vi "HFRR ADV v09.vi"() -> ()   [LabVIEW 2025] (continued)
            n4154 = property class="Instr"(reference=w5657, error in=w5636) -> (reference out=w5656:refnum<visa-resource-name>, error out=w5655:errorcluster, "Serial Settings:Number of Bytes at Serial Port"=w5654:u32)
            n4155 = Greater?(x=w5654, y=u32 100) -> (0:w5652:bool)
            n4156 = case shown="True" w5652 {
              tunnel: w5656 -> [w5695 w5720]
              tunnel: w5655 -> [w5694 w5719]
              tunnel: w5654 -> [_ w5718]
              tunnel: [w5695 w5717] -> w5642
              tunnel: [w5694 w5716] -> w5641
              tunnel: w5638 -> [w5693 w5715]
              tunnel: [w5693 ""] -> w5637
              frame False {
              }
              frame True {
                w5705 = u32 6 ("y")
                # "Page 84 of \nmanual"
                n4157 = VISA Read(VISA resource name=w5720, byte count=w5718, error in (no error)=w5719) -> (VISA resource name out=w5717:refnum<visa-resource-name>, read buffer=w5713:string, error out=w5716:errorcluster)  [unwired: 1 out]
                n4158 = while {
                  tunnel: w5713 -> [w5769]
                  tunnel: [w5765] -> w5707 mode=indexing
                  tunnel: [w5759] -> w5711 mode=indexing
                  tunnel: [w5757] -> _
                  i -> [w5757]
                  stop <- w5762 stop-if-true
                  n4159 = String Subset(string=w5769, offset (0)=w5757) -> (substring=w5764:string)  [unwired: 1 in]
                  n4160 = String To Byte Array(string=w5764) -> (unsigned byte array=w5768:u8[])
                  n4161 = String Length(string=w5764) -> (length=w5763:i32)
                  n4162 = Index Array(array=w5768) -> (element=w5767:u8)  [unwired: 1 in]
                  n4163 = Equal To 0?(x=w5763) -> (x = 0?=w5762:bool)
                  n4164 = Number To Boolean Array(number=w5767) -> (Boolean array=w5761:bool[])
                  n4165 = Reverse 1D Array(array=w5761) -> (reversed array=w5760:bool[])
                  n4166 = And(x=w5761, y=bool[] [FALSE, FALSE, FALSE, FALSE, FALSE, FALSE, TRUE, TRUE] ("Boolean array")) -> (x .and. y?=w5765:bool[])
                  n4167 = And(x=w5760, y=bool[] [FALSE, FALSE, TRUE, TRUE, TRUE, TRUE, TRUE, TRUE] ("Boolean array")) -> (x .and. y?=w5759:bool[])
                }
                n4168 = Concatenate Strings(w5715, w5713) -> (→"Read String":string)
                n4169 = while {
                  tunnel: w5707 -> [w5756] mode=indexing
                  tunnel: [w5752] -> w5710
                  i -> [w5752]
                  stop <- w5753 stop-if-true
                  n4170 = Search 1D Array(1D array=w5756, element=TRUE) -> (index of element=w5754:i32)  [unwired: 1 in]
                  n4171 = Less Than 0?(x=w5754) -> (x < 0?=w5753:bool)
                }
                n4172 = Delete From Array(array=w5711, length=w5710, index (row)=0) -> (array with subset deleted=w5706:bool[][])  [unwired: 1 in, 1 out]
                n4173 = Array Size(array=w5706) -> (size(s)=w5708:i32[])
                n4174 = Index Array(array=w5708) -> (element=w5700:i32)  [unwired: 1 in]
                n4175 = Greater?(x=w5700, y=w5705) -> (0:w5703:bool)
                n4176 = Subtract(x=w5700, y=w5705) -> (x-y=w5704:u32)
                n4177 = Select(t=w5704, s=w5703, f=u32 0) -> (s? t:f=w5701:u32)
                n4178 = while {
                  tunnel: w5706 -> [w5739]
                  tunnel: [w5741] -> w5699 mode=indexing
                  tunnel: w5701 -> [w5723]
                  i -> [w5740]
                  stop <- w5738 stop-if-true
                  w5730 = 6 ("index")
                  w5729 = 2 ("length")
                  # "Page 65 of \nmanual"
                  n4179 = Multiply(x=u32 3 ("y"), y=w5740) -> (x*y=w5737:u32)
                  n4180 = Divide(x=u32 102 ("y"), y=u32 65520) -> (x/y=w5747:dbl)
                  n4181 = Greater Or Equal?(x=w5737, y=w5723) -> (x >= y?=w5738:bool)
                  n4182 = Index Array(array=w5739, index (row) #1=w5737) -> (element #1=w5735:bool[], element #2=w5734:bool[], element #3=w5733:bool[])  [unwired: 5 in]
                  n4183 = Reverse 1D Array(array=w5735) -> (reversed array=w5728:bool[])
                  n4184 = Reverse 1D Array(array=w5734) -> (reversed array=w5732:bool[])
                  n4185 = Reverse 1D Array(array=w5733) -> (reversed array=w5731:bool[])
                  n4186 = Delete From Array(array=w5728, length=w5729, index=w5730) -> (array with subset deleted=w5724:bool[])  [unwired: 1 out]
                  n4187 = Delete From Array(array=w5732, length=w5729, index=w5730) -> (array with subset deleted=w5725:bool[])  [unwired: 1 out]
                  n4188 = Delete From Array(array=w5731, length=w5729, index=w5730) -> (array with subset deleted=w5726:bool[])  [unwired: 1 out]
                  n4189 = Insert Into Array(array=bool[] [] ("Boolean array"), new element #1=w5724, new element #2=w5725, new element #3=w5726) -> (w5727:bool[])  [unwired: 1 in]
                  n4190 = Boolean Array To Number(Boolean array=w5727) -> (number=w5736:u32)
                  n4191 = Multiply(x=w5747, y=w5736) -> (x*y=w5746:dbl)
                  n4192 = Decrement(x=w5746) -> (x-1=w5745:dbl)
                  n4193 = Divide(x=w5745, y=u32 100) -> (x/y=w5743:dbl)
                  n4194 = Multiply(x=w5743, y=u32 10) -> (x*y=w5741:dbl)
                }
                n4195 = Delete From Array(array=w5699) -> (array with subset deleted=w5698:dbl[])  [unwired: 2 in, 1 out]
                "Waveform Graph 5" <- w5698
                "Waveform Chart 3" <- w5698
                n4196 = call-poly <vilib>:"Mean.vi"("X"=w5698) -> ("mean"=w5697:dbl)  [unwired: 1 out]
                "Measure_LDS" <- w5697
                n4197 = case shown="True" "Zero 4" {
                  tunnel: w5697 -> [_ w5722]
                  frame False {
                  }
                  frame True {
                    n4198 = local write "Zero 4"(FALSE ("Zero 4")) -> ()
                    "z_measure" <- w5722
                  }
                }
              }
            }
            n4199 = local read "Measure_LDS"() -> (w5632:dbl)
            n4200 = local read "Disp (mm)"() -> (w5631:dbl)
            n4201 = local read "Boolean 7"() -> (w5630:bool)
            n4202 = local read "Boolean 8"() -> (w5629:bool)
            n4203 = case shown="True" "Boolean 8" {
              tunnel: w5631 -> [_ w5662]
              tunnel: w5632 -> [_ w5661]
              frame False {
              }
              frame True {
                n4204 = local read "Captured Values 2"() -> (w5665:dbl[][])
                n4205 = Build Array(w5662, w5661) -> (w5660:dbl[])
                n4206 = Build Array (concatenate)(w5665, w5660) -> (w5663:dbl[][])
                n4207 = local write "Captured Values 2"(w5663) -> ()
                n4208 = local write "Boolean 8"(FALSE ("Boolean 8")) -> ()
              }
            }
            n4209 = call "Build XY Graph"("Enable"=w5629, "Reset"=w5630, "Y Input"=w5632, "X Input"=w5631) -> ("XY Graph"=→"?":cluster{"Y":dbl[], "Y":dbl[]}[])  [unwired: 6 in, 1 out]
            n4210 = case shown="True" "Boolean 9" {
              frame False {
              }
              frame True {
                n4211 = local read "Captured Values 2"() -> (w5667:dbl[][])
                n4212 = Index Array(array=w5667, index (col) #1=0 ("disabled index (col)"), index (col) #2=1 ("index (col)")) -> (element #1=w5670:dbl[], element #2=w5669:dbl[])  [unwired: 2 in]
                n4213 = call <vilib>:"Linear Fit.vi"("Y"=w5670, "X"=w5669) -> ("slope"=→"Slope":dbl, "intercept"=→"Intercept":dbl)  [unwired: 9 in, 3 out]
                n4214 = local write "Boolean 9"(FALSE ("Boolean 9")) -> ()
              }
            }
            n4215 = case shown="True" "Boolean 7" {
              frame False {
              }
              frame True {
                n4216 = local write "Captured Values 2"(dbl[][] [] ("Captured Values")) -> ()
                n4217 = local write "Boolean 7"(FALSE ("Boolean 7")) -> ()
              }
            }
            n4218 = Concatenate Strings("COMMAND 2", "\r", "\n") -> (w5644:string)
            n4219 = case shown="True" "Measure 2" {
              tunnel: w5642 -> [w5677 w5683]
              tunnel: w5641 -> [w5676 w5682]
              tunnel: [w5677 w5681] -> w5640
              tunnel: [w5676 w5680] -> w5639
              tunnel: w5644 -> [_ w5679]
              frame False {
              }
              frame True {
                n4220 = local write "Measure 2"(FALSE ("WRITE")) -> ()
                n4221 = VISA Write(VISA resource name=w5683, write buffer=w5679, error in (no error)=w5682) -> (VISA resource name out=w5681:refnum<visa-resource-name>, error out=w5680:errorcluster)  [unwired: 1 out]
              }
            }
          }
          frame Error {
            w5772 = u16 10 items=["1.0"=10, "1.5"=15, "2.0"=20] ("stop bits (10: 1 bit)")
            n4222 = Wait (ms)(milliseconds to wait=u32 20) -> ()  [unwired: 1 out]
            n4223 = VISA Close(VISA resource name=w5774, error in (no error)=w5780) -> (error out=w5779:errorcluster)
            n4224 = call <vilib>:"Clear Errors.vi"("error in (no error)"=w5779) -> ("error out"=w5778:errorcluster)  [unwired: 5 in, 1 out]
            n4225 = call-poly "VISA Configure Serial Port"("VISA resource name"="Laser Disp Sensor", "timeout (10sec)"=u32 200, "Enable Termination\nChar (T)"=TRUE ("Enable Termination\nChar (T)"), "baud rate (9600)"=u32 921600, "error in (no error)"=w5778, "stop bits (10: 1 bit)"=w5772) -> ("VISA resource name out"=w5782:refnum<visa-resource-name>, "error out"=w5781:errorcluster)  [unwired: 8 in]
          }
        }
        n4226 = local read "Quit"() -> (w5616:bool)
      }
      n4227 = VISA Close(VISA resource name=w5611, error in (no error)=w5612) -> (error out=w5610:errorcluster)
      n4228 = call <vilib>:"Clear Errors.vi"("error in (no error)"=w5610) -> ()  [unwired: 5 in, 2 out]
    }
    frame Enabled {
    }
  }
  n4229 = disable-structure shown="Disabled" {
    disable-tunnel: _ -> [w5787 _]
    frame Disabled {
      n4230 = while {
        tunnel: [w5794] -> _
        shift-right: [w5791] -> w5784
        shift-left: _ -> [w5793]
        shift-right: [w5792] -> w5785
        shift-left: errorcluster {"status"=TRUE, "code"=0, "source"="Init"} ("error out") -> [w5790]
        tunnel: w5787 -> [_]
        i -> [w5794]
        stop <- w5788 stop-if-true
        n4231 = flat-sequence {
          tunnel: w5790 -> [w5885]
          tunnel: [w5885] -> w5789
          frame #0 {
            n4232 = Wait (ms)(milliseconds to wait=u32 50) -> ()  [unwired: 1 out]
          }
        }
        n4233 = case shown="No Error" w5789 {
          selector: w5789 -> [w5835 w5878]
          tunnel: w5793 -> [w5834 w5877]
          tunnel: [w5801 w5868] -> w5792
          tunnel: [w5802 w5876] -> w5791
          frame No Error {
            w5828 = T28 {"Mode"=enum."RTU", "Slave Address"=1} ("Serial Parameters")
            n4234 = call-poly <vilib>:"MB Serial Master Query (poly).vi"("VISA resource name"=w5834, "Starting Address"=i16 1000, "Quantity"=u16 1, "Timeout"=u32 1000, "error in"=w5835, "Serial Parameters"=w5828) -> ("VISA resource name out"=w5829:refnum<visa-resource-name>, "Input Registers"=w5831:u16[], "error out"=w5827:errorcluster)  [unwired: 10 in, 1 out]
            n4235 = Random Number (0-1)() -> (number: 0 to 1=w5816:dbl)
            n4236 = Index Array(array=w5831, index=0) -> (element=w5826:u16)
            n4237 = Subtract(x=w5816, y=0.5) -> (x-y=w5815:dbl)
            n4238 = Divide(x=w5826, y=10 ("index")) -> (x/y=w5820:dbl)
            n4239 = Multiply(x=w5815, y=0.5) -> (x*y=w5814:dbl)
            n4240 = Add(x=w5820, y=w5814) -> (x+y=w5819:dbl)
            n4241 = local read "Amb temp"() -> (w5803:dbl)
            n4242 = Multiply(x=w5819, y=0.2) -> (x*y=w5823:dbl)
            n4243 = Multiply(x=w5803, y=0.8) -> (x*y=w5821:dbl)
            n4244 = Add(x=w5823, y=w5821) -> (x+y=w5804:dbl)
            n4245 = local read "set temp old"() -> (w5798:dbl)
            n4246 = local write "Amb temp"(w5804) -> ()
            n4247 = Select(t="SetTemp 2", s="Heater", f=100.0) -> (s? t:f=w5799:dbl)
            n4248 = Not Equal?(x=w5799, y=w5798) -> (x != y?=w5797:bool)
            n4249 = case shown="True" w5797 {
              tunnel: w5829 -> [w5863 w5865]
              tunnel: [w5862 w5865] -> w5809
              tunnel: w5827 -> [w5861 w5864]
              tunnel: [w5860 w5864] -> w5807
              tunnel: w5799 -> [w5855 _]
              tunnel: w5828 -> [w5857 w5866]
              tunnel: [w5857 w5866] -> w5810
              frame True {
                n4250 = Multiply(x=w5855, y=10 ("index")) -> (x*y=w5854:dbl)
                n4251 = call-poly <vilib>:"MB Serial Master Query (poly).vi"("VISA resource name"=w5863, "Address"=u16 0, "Holding Register"=w5854, "Timeout"=u32 1000, "error in"=w5861, "Serial Parameters"=w5857) -> ("VISA resource name out"=w5862:refnum<visa-resource-name>, "error out"=w5860:errorcluster)  [unwired: 11 in, 1 out]
                "set temp old" <- w5855
              }
              frame False {
              }
            }
            n4252 = flat-sequence {
              tunnel: [w5836] -> _
              tunnel: [w5836] -> w5806
              tunnel: w5807 -> [w5836]
              frame #0 {
                n4253 = Wait (ms)(milliseconds to wait=u32 100) -> ()  [unwired: 1 out]
              }
            }
            n4254 = call "Elapsed Time12"("Time Target (s)"=2.0, "Auto Reset"=TRUE) -> ("Time has Elapsed"=w5811:bool)  [unwired: 10 in, 7 out]
            n4255 = case shown="True" w5811 {
              tunnel: w5810 -> [w5840 w5853]
              tunnel: [w5840 w5853] -> _
              tunnel: [w5839 w5851] -> w5802
              tunnel: w5809 -> [w5839 w5852]
              tunnel: [w5838 w5849] -> w5801
              tunnel: w5806 -> [w5838 w5850]
              frame False {
              }
              frame True {
                n4256 = call-poly <vilib>:"MB Serial Master Query (poly).vi"("VISA resource name"=w5852, "Starting Address"=i16 1003 ("Addr"), "Quantity"=u16 1, "Timeout"=u32 1000, "error in"=w5850, "Serial Parameters"=w5853) -> ("VISA resource name out"=w5851:refnum<visa-resource-name>, "Input Registers"=w5846:u16[], "error out"=w5849:errorcluster)  [unwired: 10 in, 1 out]
                n4257 = Index Array(array=w5846, index=0) -> (element=w5845:u16)
                n4258 = Divide(x=w5845, y=u16 10) -> (x/y=w5841:dbl)
                n4259 = local write "set temp old"(w5841) -> ()
                n4260 = local write "SetTemp"(w5841) -> ()
              }
            }
            "Error Code" <- w5801
            n4261 = Unbundle(w5801) -> ("status"=→"TK4 status":bool)  [unwired: 2 out]
            "SetTemp" <- "SetTemp 2"
          }
          frame Error {
            w5880 = u16 0 items=["None", "Odd", "Even", "Mark", "Space"] ("Parity")
            w5881 = u16 0 items=["None", "XON/XOFF", "RTS/CTS", "XON/XOFF & RTS/CTS", "DTR/DSR", "XON/XOFF & DTR/DSR"] ("Flow Control")
            n4262 = VISA Clear(VISA resource name=w5877, error in (no error)=w5878) -> (VISA resource name out=w5871:refnum<visa-resource-name>, error out=w5869:errorcluster)
            n4263 = VISA Close(VISA resource name=w5871, error in (no error)=w5869) -> (error out=w5870:errorcluster)
            n4264 = call <vilib>:"Clear Errors.vi"("error in (no error)"=w5870) -> ("error out"=w5879:errorcluster)  [unwired: 5 in, 1 out]
            n4265 = Unbundle By Name(T28 {"Mode"=enum."RTU", "Slave Address"=1} ("input cluster")) -> ("Mode"=w5882:enum16{"RTU", "ASCII"})
            n4266 = call <vilib>:"MB Serial Init.vi"("Timeout"=u32 100, "Flow Control"=w5881, "Mode"=w5882, "error in (no error)"=w5879, "Parity"=w5880, "Baud Rate"=u32 9600, "VISA resource name"="Lubrication System COM Port :") -> ("error out"=w5868:errorcluster, "VISA resource name out"=w5876:refnum<visa-resource-name>)  [unwired: 3 in]
            n4267 = local write "set temp old"(0.0 ("set temp old")) -> ()
            n4268 = Unbundle(w5868) -> ("status"=w5867:bool)  [unwired: 2 out]
            n4269 = case shown="True" w5867 {
              selector: w5867 -> [_ w5884]
              frame False {
              }
              frame True {
                n4270 = local write "TK4 status"(w5884) -> ()
              }
            }
          }
        }
        n4271 = local read "Quit"() -> (w5788:bool)
      }
      n4272 = VISA Close(VISA resource name=w5784, error in (no error)=w5785) -> (error out=w5783:errorcluster)
      n4273 = call <vilib>:"Clear Errors.vi"("error in (no error)"=w5783) -> ()  [unwired: 5 in, 2 out]
    }
    frame Enabled {
    }
  }
  "file count" <- 0 ("file count")
